vi "Create Ball Joint.vi"(9 "Radius 2":sgl=0.5, 10 "Name":string="MachineBase", 11 "RGBA":cluster{"R":sgl, "G":sgl, "B":sgl, "A":sgl}) -> (1 "Transformation.GetTranslation":T1, 3 "SceneObject out":refnum<vi>)   [LabVIEW 2021]
uses:
  <vilib>/Utility/miscctls.llb/LV3DPointTypeDef.ctl
  <vilib>/picture/3D Picture Control/Object/Create Object (drawable).vi
  <vilib>/picture/3D Picture Control/NI_3D Picture Control.lvlib
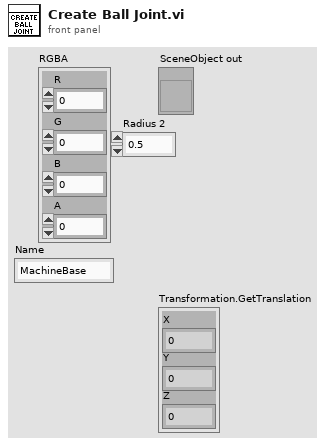
[diagram p1: front panel]
types:
  T1 = typedef "LV3DPointTypeDef.ctl" = cluster{"X":sgl, "Y":sgl, "Z":sgl}
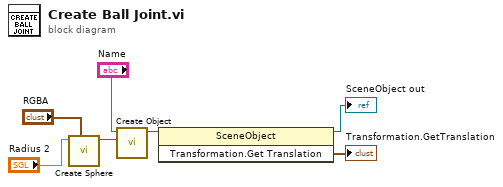
[diagram p0: block diagram]
diagram:
  n1 = call <vilib>:"Create Sphere.vi"("Color"="RGBA", "Radius"="Radius 2") -> ("New Sphere Refnum"=w2:refnum<vi>)  [unwired: 8 in, 1 out]
  n2 = call-poly <vilib>:"Create Object.vi"("Geometry"=w2, "Name"="Name") -> ("Scene:New Object"=w3:refnum<vi>)  [unwired: 8 in, 1 out]
  n3 = invoke class="SceneObject" method="Transformation.Get Translation"(reference=w3) -> (reference out=→"SceneObject out":refnum<vi>, "Transformation.GetTranslation"=→"Transformation.GetTranslation":T1)  [unwired: 2 in, 1 out]
